vi "Tmp_M connect to simulated device.vi"(8 "error in (no error)":errorcluster, 11 "VISA Refnum in":refnum<visa-resource-name>) -> (0 "error out":errorcluster, 2 "TM Revision":T1, 3 "VISA Refnum out":refnum<visa-resource-name>)   [LabVIEW 2017, in "Magnet module.lvlib"]
doc: "Initialize comunication with Temperature Monitor and gets its revision info. At least model name should be send as message to master module."
uses:
  Magnet module.lvlib
  ctl/TM Revision.ctl
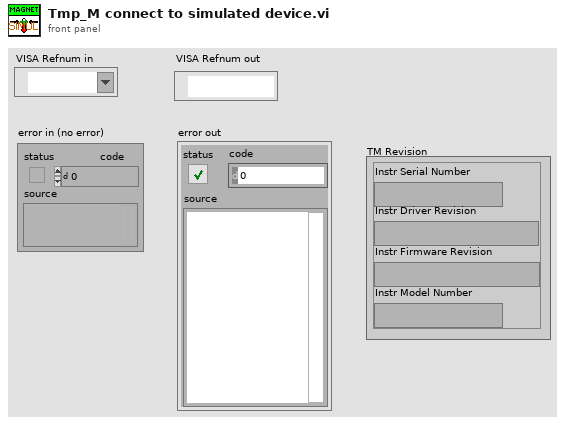
[diagram p1: front panel]
types:
  T1 = typedef "Magnet module.lvlib/TM Revision.ctl" = cluster{"Instr Serial Number":string, "Instr Driver Revision":string, "Instr Firmware Revision":string, "Instr Model Number":string}
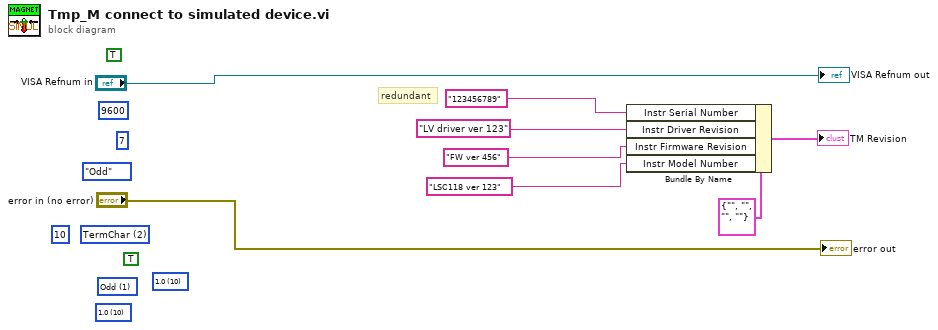
[diagram p0: block diagram]
diagram:
  (unwired) u16 10 items=["1.0"=10, "1.5"=15, "2.0"=20] ("Serial Settings:Stop Bits")
  (unwired) u16 1 items=["None", "Odd", "Even", "Mark", "Space"] ("Serial Settings:Parity")
  (unwired) TRUE ("Message Based Settings:Send End Enable")
  (unwired) u16 2 items=["None", "Last Bit", "TermChar", "Break"] ("Serial Settings:End Mode for Writes")
  (unwired) TRUE ("Enable Termination\nChar (T)")
  (unwired) u16 7 ("data bits (8)")
  (unwired) u32 9600 ("baud rate (9600)")
  (unwired) enum16{"None", "Odd", "Even", "Mark", "Space"}."Odd" ("parity (0:none)")
  (unwired) u16 10 items=["1.0"=10, "1.5"=15, "2.0"=20] ("stop bits (10: 1 bit)")
  (unwired) u8 10 ("termination char\n(0xA = '\\n' = LF)")
  # "redundant"
  n1 = Bundle By Name(cluster=T1 {"Instr Serial Number"="", "Instr Driver Revision"="", "Instr Firmware Revision"="", "Instr Model Number"=""} ("Revision"), "Instr Serial Number"="123456789", "Instr Driver Revision"="LV driver ver 123" ("Instr Serial Number"), "Instr Firmware Revision"="FW ver 456" ("Instr Serial Number"), "Instr Model Number"="LSC118 ver 123" ("Instr Serial Number")) -> (→"TM Revision":T1)
  "error out" <- "error in (no error)"
  "VISA Refnum out" <- "VISA Refnum in"
